vi "Lidar Loop.vi"() -> (2 "Lidar Run Time":u32, 3 "XY Graph":cluster{"X":dbl[], "Y":dbl[]}[](graph))   [LabVIEW 2018]
uses:
  Control Globals.vi
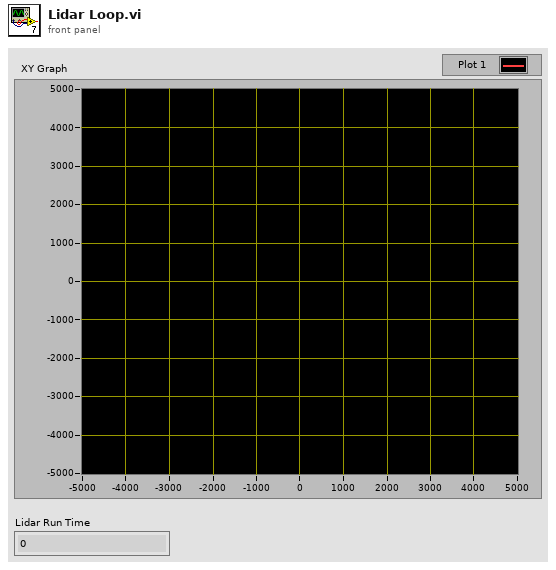
[diagram p1: front panel]
types:
  T1 = cluster{"X":dbl[], "Y":dbl[], "Estimated Pose":cluster{"X":dbl, "Y":dbl, "R":dbl}}
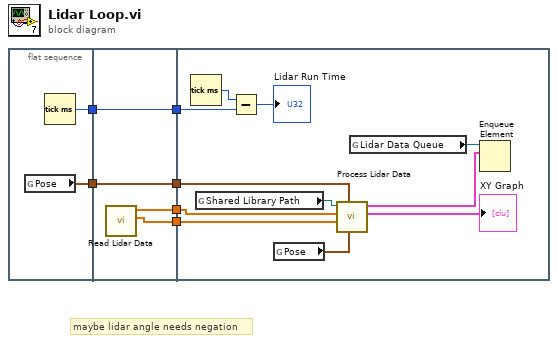
[diagram p0: block diagram]
diagram:
  # "maybe lidar angle needs negation"
  n1 = flat-sequence {
    tunnel: [w8] -> w6
    tunnel: [w7] -> w5
    tunnel: [w12] -> w4
    tunnel: [w11] -> w3
    tunnel: [w10] -> w2
    tunnel: w6 -> [w10]
    tunnel: [w9] -> w1
    tunnel: w5 -> [w9]
    tunnel: w4 -> [w20]
    tunnel: w3 -> [w21]
    tunnel: w2 -> [w23]
    tunnel: w1 -> [w16]
    frame #0 {
      n2 = global read "Control Globals.vi" "Pose"() -> (w8:cluster{"X":dbl, "Y":dbl, "R":dbl})
      n3 = Tick Count (ms)() -> (millisecond timer value=w7:u32)
    }
    frame #1 {
      n4 = call "Read Lidar Data.vi"() -> ("Direction"=w11:dbl[], "Magnitude"=w12:dbl[])  [unwired: 9 in, 1 out]
    }
    frame #2 {
      n5 = Tick Count (ms)() -> (millisecond timer value=w17:u32)
      n6 = global read "Control Globals.vi" "Shared Library Path"() -> (w14:path)
      n7 = Subtract(x=w17, y=w16) -> (x-y=→"Lidar Run Time":u32)
      n8 = global read "Control Globals.vi" "Pose"() -> (w15:cluster{"X":dbl, "Y":dbl, "R":dbl})
      n9 = call "Process Lidar Data.vi"("Estimated Pose After Scan"=w15, "Estimated Pose Before Scan"=w23, "Direction"=w21, "Magnitude"=w20, "path in"=w14) -> ("Data Comparison"=→"XY Graph":cluster{"X":dbl[], "Y":dbl[]}[], "Lidar Scan"=w22:T1)  [unwired: 5 in]
      n10 = global read "Control Globals.vi" "Lidar Data Queue"() -> (w13:refnum<queue>)
      n11 = Enqueue Element(queue=w13, element=w22) -> ()  [unwired: 2 in, 3 out]
    }
  }
